vi "generate random string.vi"(10 "Number of Characters":i32) -> (2 "string":string)   [LabVIEW 2015, in "E2E Tag Exchange tests.lvlib"]
uses:
  E2E Tag Exchange tests.lvlib
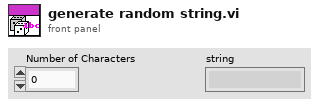
[diagram p1: front panel]
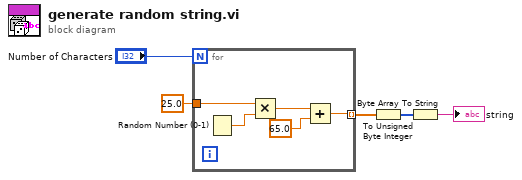
[diagram p0: block diagram]
diagram:
  n1 = for {
    N: "Number of Characters" -> [_]
    tunnel: 25.0 -> [w7]
    tunnel: [w6] -> w3 mode=indexing
    n2 = Random Number (0-1)() -> (number: 0 to 1=w10:dbl)
    n3 = Multiply(x=w7, y=w10) -> (x*y=w8:dbl)
    n4 = Add(x=w8, y=65.0) -> (x+y=w6:dbl)
  }
  n5 = To Unsigned Byte Integer(number=w3) -> (unsigned 8bit integer=w5:u8[])
  n6 = Byte Array To String(unsigned byte array=w5) -> (string=→"string":string)
